vi "Get_Target_Info.vi"(8 "Height":T1, 9 "Target Location":cluster{"X (Pixels)":dbl, "Y (Pixels)":dbl}, 10 "Resolution":cluster{"H (pixels)":dbl, "V (Pixels)":dbl}, 11 "FOV":cluster{"X (degrees)":dbl, "Y (degrees)":dbl}) -> (0 "Distance (lateral)":dbl, 1 "Distance (CT)":dbl, 2 "Elevation Delta":dbl, 3 "Yaw Delta":dbl)   [LabVIEW 2016]
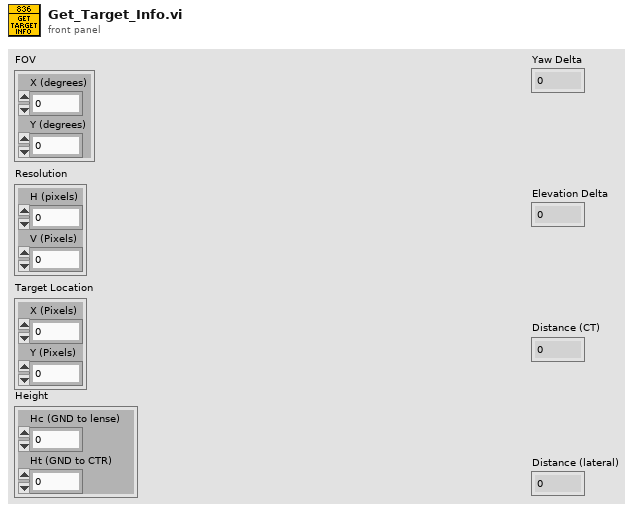
[diagram p1: front panel]
types:
  T1 = cluster{"Hc (GND to lense)":dbl, "Ht (GND to CTR)":dbl}
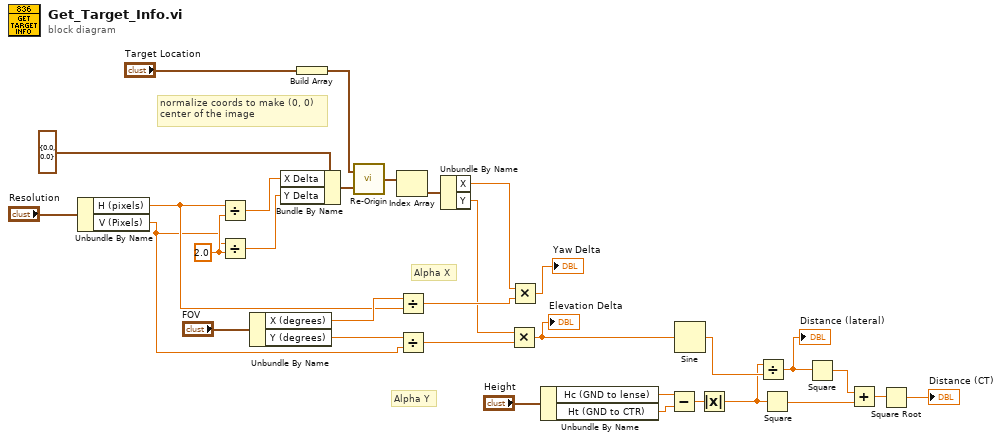
[diagram p0: block diagram]
diagram:
  w28 = 2.0 ("y")
  # "Alpha Y"
  # "Alpha X"
  # "normalize coords to make (0, 0)\ncenter of the image"
  n1 = Unbundle By Name("Resolution") -> ("H (pixels)"=w22:dbl, "V (Pixels)"=w17:dbl)
  n2 = Divide(x=w22, y=w28) -> (x/y=w27:dbl)
  n3 = Divide(x=w17, y=w28) -> (x/y=w26:dbl)
  n4 = Unbundle By Name("FOV") -> ("X (degrees)"=w23:dbl, "Y (degrees)"=w21:dbl)
  n5 = Bundle By Name(cluster=cluster{"X Delta":dbl, "Y Delta":dbl} {"X Delta"=0.0, "Y Delta"=0.0} ("Transition"), "X Delta"=w27, "Y Delta"=w26) -> (w25:cluster{"X Delta":dbl, "Y Delta":dbl})
  n6 = Build Array("Target Location") -> (w30:cluster{"X (Pixels)":dbl, "Y (Pixels)":dbl}[])
  n7 = call "Re-Origin.vi"("Transition"=w25, "Coordinates"=w30) -> ("Normalized Coords"=w19:cluster{"X":dbl, "Y":dbl}[])
  n8 = Index Array(array=w19) -> (element=w18:cluster{"X":dbl, "Y":dbl})  [unwired: 1 in]
  n9 = Divide(x=w23, y=w22) -> (x/y=w20:dbl)
  n10 = Divide(x=w21, y=w17) -> (x/y=w16:dbl)
  n11 = Unbundle By Name(w18) -> ("X"=w15:dbl, "Y"=w14:dbl)
  n12 = Multiply(x=w14, y=w16) -> (x*y=w12:dbl)
  "Elevation Delta" <- w12
  n13 = Multiply(x=w15, y=w20) -> (x*y=→"Yaw Delta":dbl)
  n14 = Unbundle By Name("Height") -> ("Hc (GND to lense)"=w10:dbl, "Ht (GND to CTR)"=w9:dbl)
  n15 = Subtract(x=w10, y=w9) -> (x-y=w8:dbl)
  n16 = Sine(x=w12) -> (sin(x)=w7:dbl)
  n17 = Absolute Value(x=w8) -> (abs(x)=w5:dbl)
  n18 = Divide(x=w5, y=w7) -> (x/y=w6:dbl)
  "Distance (lateral)" <- w6
  n19 = Square(x=w5) -> (x^2=w3:dbl)
  n20 = Square(x=w6) -> (x^2=w4:dbl)
  n21 = Add(x=w4, y=w3) -> (x+y=w2:dbl)
  n22 = Square Root(x=w2) -> (sqrt(x)=→"Distance (CT)":dbl)
